vi "Enable UI.vi"(8 "error in (no error)":errorcluster, 11 "Server UI in":refnum<class "Server UI.lvclass">) -> (0 "error out":errorcluster, 3 "Server UI out":refnum<class "Server UI.lvclass">)   [LabVIEW 2016, in "Server UI.lvlib" / "Server UI.lvclass"]
uses:
  Server UI.lvclass
  Server UI.lvclass/Server UI.ctl
  Read Start Server.vi
  MAL-Framework/user.lib/Common Components/Msmt UI/Measurement UI.lvclass
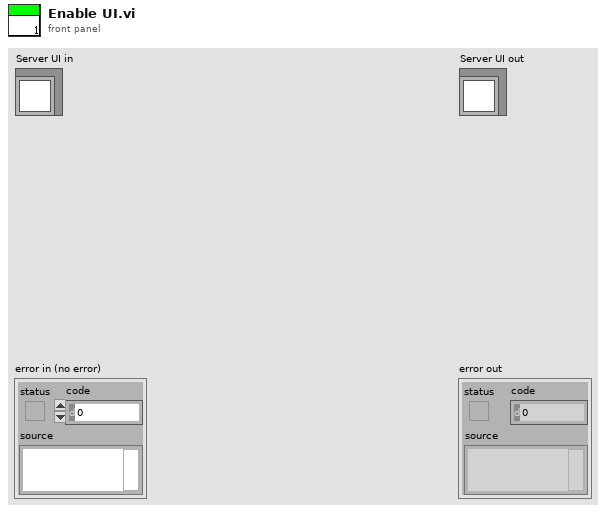
[diagram p1: front panel]
types:
  T1 = enum8{"Enabled", "Disabled", "Disabled and Grayed Out"}
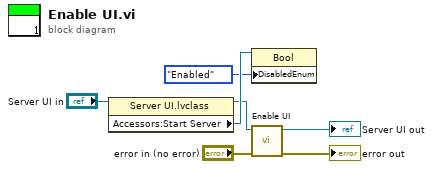
[diagram p0: block diagram]
diagram:
  n1 = property class="Server UI.lvclass"(reference="Server UI in") -> (reference out=w2:refnum<class "Server UI.lvclass">, "Accessors:Start Server"=w3:refnum<vi>)  [unwired: 1 in, 1 out]
  n2 = property class="Bool"(reference=w3, "DisabledEnum"=T1."Enabled" ("Disabled")) -> ()  [unwired: 1 in, 2 out]
  n3 = call-parent "Enable UI.vi"("error in (no error)"="error in (no error)", "Measurement UI in"=w2) -> ("error out"=→"error out":errorcluster, "Measurement UI out"=→"Server UI out":refnum<class "Server UI.lvclass">)  [unwired: 8 in]
